vi "CTRE_CANifier_GetGeneralInputs.vi"(8 "error in":errorcluster, 11 "CANifierDevRef":T2) -> (0 "error out":errorcluster, 2 "General IO Pins":T1={"QUAD_IDX"=TRUE, "QUAD_B"=TRUE, "QUAD_A"=TRUE, "LIMR"=TRUE, "LIMF"=TRUE, "SDA"=TRUE, "SCL"=TRUE, "SPI_CS"=TRUE, "SPI_MISO_PWM2"=TRUE, "SPI_MOSI_PWM1"=TRUE, "SPI_CLK_PWM0"=TRUE}, 3 "CANifierDevRef":T2)   [LabVIEW 2016]
uses:
  <vilib>/Rock Robotics/WPI/ThirdParty/Sensors/CANifier/CTRE_CANifier_DeviceRef.ctl
  <vilib>/Rock Robotics/WPI/ThirdParty/Sensors/CANifier/CTRE_CANifier_GeneralPinsCluster.ctl
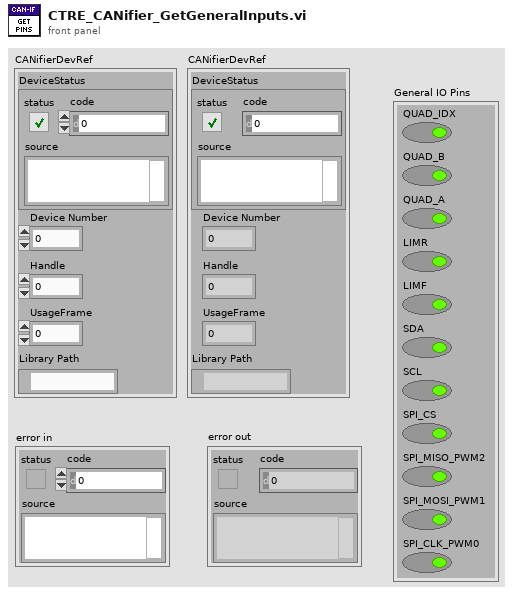
[diagram p1: front panel]
types:
  T1 = typedef "CTRE_CANifier_GeneralPinsCluster.ctl" = cluster{"QUAD_IDX":bool, "QUAD_B":bool, "QUAD_A":bool, "LIMR":bool, "LIMF":bool, "SDA":bool, "SCL":bool, "SPI_CS":bool, "SPI_MISO_PWM2":bool, "SPI_MOSI_PWM1":bool, "SPI_CLK_PWM0":bool}
  T2 = typedef "CTRE_CANifier_DeviceRef.ctl" = cluster{"DeviceStatus":errorcluster, "Device Number":u8, "Handle":u64, "UsageFrame":u32, "Library Path":path}
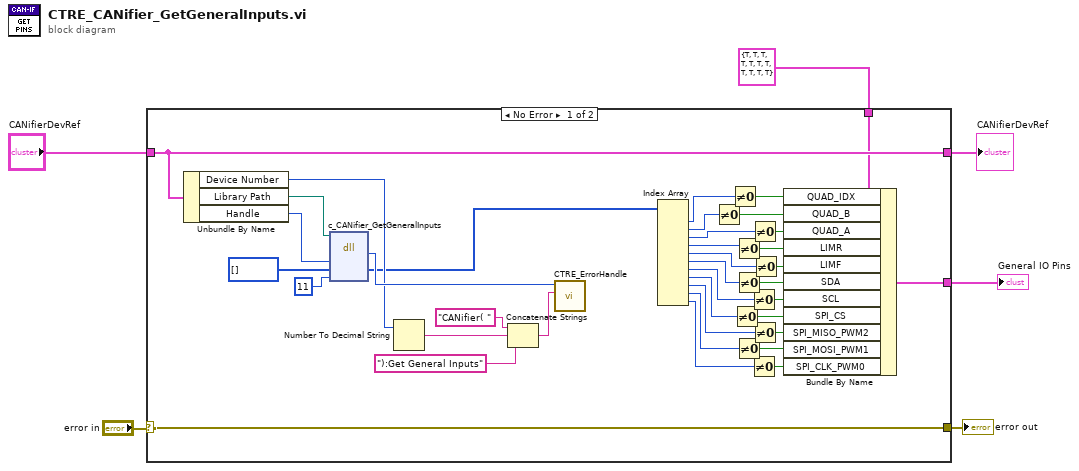
[diagram p0: block diagram]
diagram:
  n1 = case shown="No Error" "error in" {
    selector: "error in" -> [w43 w45]
    tunnel: [w43 w45] -> w5
    tunnel: "CANifierDevRef" -> [w42 w44]
    tunnel: [w42 w44] -> w3
    tunnel: T1 {"QUAD_IDX"=TRUE, "QUAD_B"=TRUE, "QUAD_A"=TRUE, "LIMR"=TRUE, "LIMF"=TRUE, "SDA"=TRUE, "SCL"=TRUE, "SPI_CS"=TRUE, "SPI_MISO_PWM2"=TRUE, "SPI_MOSI_PWM1"=TRUE, "SPI_CLK_PWM0"=TRUE} ("General IO Pins 2") -> [w31 _]
    tunnel: [w30 _] -> w1
    frame No Error {
      n2 = Unbundle By Name(w42) -> ("Device Number"=w35:u8, "Library Path"=w41:path, "Handle"=w40:u64)
      n3 = dll-call lib="?" fn="c_CANifier_GetGeneralInputs"(path in=w41, "handle"=w40, "allPins"=u8[] [], "capacity"=u8 11) -> ("CTR_Code"=w39:i8, "allPins"=w28:u8[])  [unwired: 4 in, 2 out]
      n4 = Number To Decimal String(number=w35) -> (decimal integer string=w38:string)  [unwired: 1 in]
      n5 = Concatenate Strings("CANifier( " ("string"), w38, "):Get General Inputs" ("string")) -> (w34:string)
      n6 = call <vilib>:"CTRE_ErrorHandle.vi"("origin"=w34, "code"=w39) -> ()  [unwired: 9 in, 1 out]
      n7 = Index Array(array=w28) -> (element #1=w27:u8, element #2=w25:u8, element #3=w23:u8, element #4=w21:u8, element #5=w19:u8, element #6=w17:u8, element #7=w15:u8, element #8=w13:u8, element #9=w11:u8, element #10=w9:u8, element #11=w7:u8)  [unwired: 11 in]
      n8 = Not Equal To 0?(x=w25) -> (x != 0?=w26:bool)
      n9 = Not Equal To 0?(x=w27) -> (x != 0?=w29:bool)
      n10 = Not Equal To 0?(x=w13) -> (x != 0?=w14:bool)
      n11 = Not Equal To 0?(x=w21) -> (x != 0?=w22:bool)
      n12 = Not Equal To 0?(x=w17) -> (x != 0?=w18:bool)
      n13 = Not Equal To 0?(x=w9) -> (x != 0?=w10:bool)
      n14 = Not Equal To 0?(x=w15) -> (x != 0?=w16:bool)
      n15 = Not Equal To 0?(x=w7) -> (x != 0?=w8:bool)
      n16 = Not Equal To 0?(x=w23) -> (x != 0?=w24:bool)
      n17 = Not Equal To 0?(x=w11) -> (x != 0?=w12:bool)
      n18 = Not Equal To 0?(x=w19) -> (x != 0?=w20:bool)
      n19 = Bundle By Name(cluster=w31, "QUAD_IDX"=w29, "QUAD_B"=w26, "QUAD_A"=w24, "LIMR"=w22, "LIMF"=w20, "SDA"=w18, "SCL"=w16, "SPI_CS"=w14, "SPI_MISO_PWM2"=w12, "SPI_MOSI_PWM1"=w10, "SPI_CLK_PWM0"=w8) -> (w30:T1)
    }
    frame Error {
    }
  }
  "error out" <- w5
  "CANifierDevRef" <- w3
  "General IO Pins" <- w1
